vi "Pinout.vi"() -> (1 "Out":T1={"LEWO"=7, "PRAWO"=11, "GÓRA"=35, "Dӣ"=36, "CZUJNIK"=12})   [LabVIEW 2014]
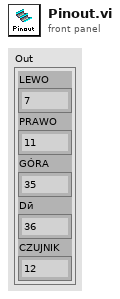
[diagram p1: front panel]
types:
  T1 = cluster{"LEWO":u8, "PRAWO":u8, "GÓRA":u8, "Dӣ":u8, "CZUJNIK":u8}
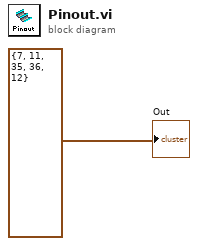
[diagram p0: block diagram]
diagram:
  "Out" <- T1 {"LEWO"=7, "PRAWO"=11, "GÓRA"=35, "Dӣ"=36, "CZUJNIK"=12} ("Cluster")
